vi "cDAQcoverterfilereader.vi"(8 "error in (no error)":errorcluster, 11 "name or relative path":string="Settings\\cDAQ\\converterSettings.txt") -> (0 "error out":errorcluster, 1 "Range":dbl[](array[numeric]), 2 "AI Max range of cDAQ":dbl[](array[numeric]), 3 "AI Min range of cDAQ":dbl[](array[numeric]), 5 "offset":dbl[](array[numeric]))   [LabVIEW 2019]
uses:
  <vilib>/Utility/file.llb/Read Delimited Spreadsheet (string).vi
panel:
  out "all rows":string[][](array[string])
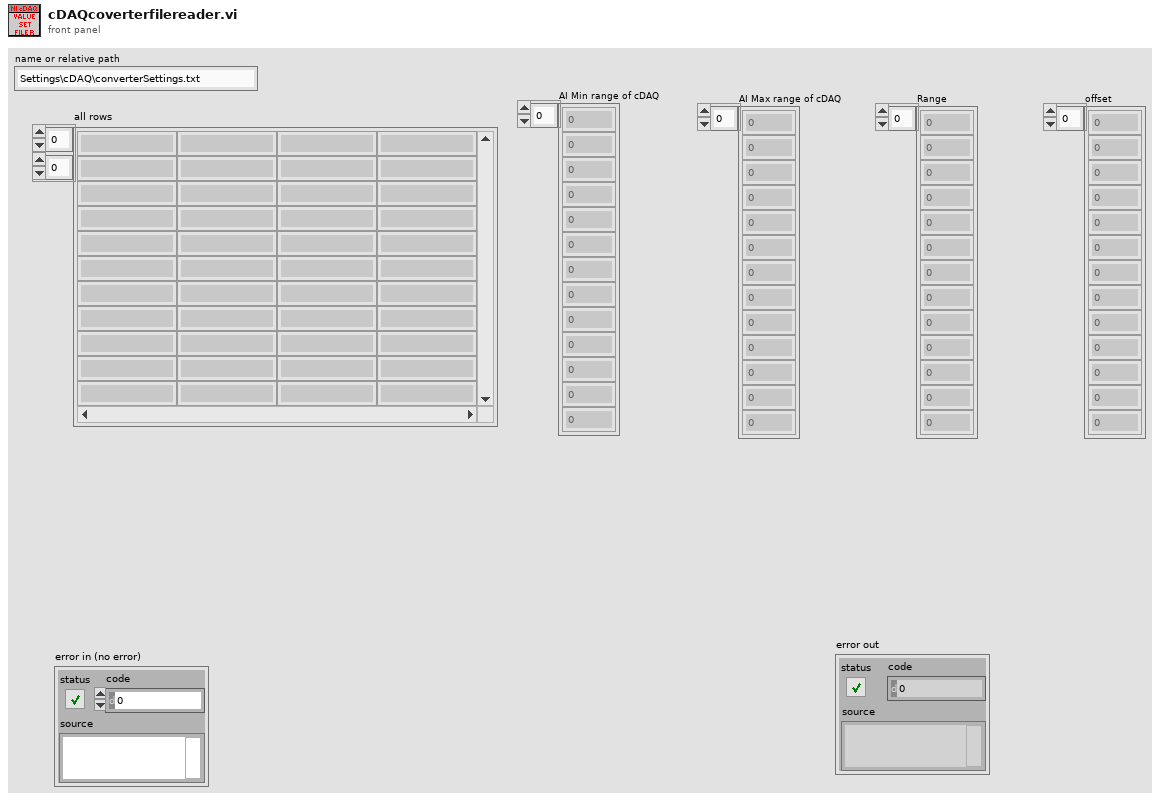
[diagram p1: front panel]
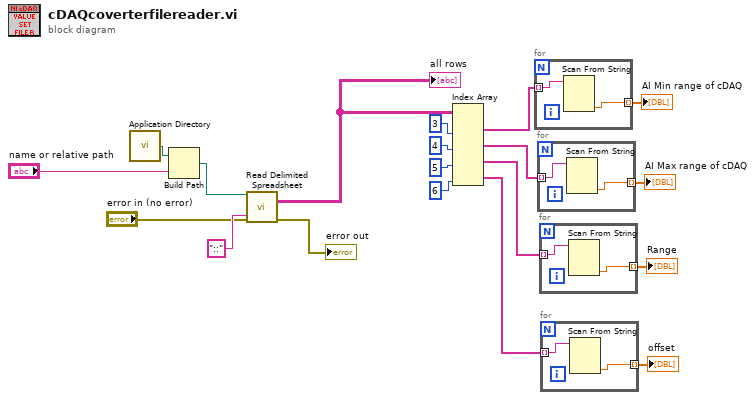
[diagram p0: block diagram]
diagram:
  n1 = call <vilib>:"Application Directory.vi"() -> ("Application Directory"=w19:path)
  n2 = Build Path(base path=w19, name or relative path="name or relative path") -> (appended path=w17:path)
  n3 = call-poly <vilib>:"Read Delimited Spreadsheet.vi"("file path (dialog if empty)"=w17, "error in (no error)"="error in (no error)", "delimiter (\\t)"="::" ("format (%.3f)")) -> ("all rows"=w15:string[][], "error out"=→"error out":errorcluster)  [unwired: 7 in, 4 out]
  "all rows" <- w15
  n4 = Index Array(array=w15, index (col) #1=3 ("disabled index (col)"), index (col) #2=4 ("index (col)"), index (col) #3=5 ("index (col)"), index (col) #4=6 ("index (col)")) -> (element #1=w9:string[], element #2=w8:string[], element #3=w7:string[], element #4=w1:string[])  [unwired: 4 in]
  n5 = for {
    tunnel: w9 -> [w21] mode=indexing
    tunnel: [w20] -> w6 mode=indexing
    n6 = Scan From String(input string=w21) -> (output 1=w20:dbl)  [unwired: 4 in, 3 out]
  }
  "AI Min range of cDAQ" <- w6
  n7 = for {
    tunnel: w8 -> [w23] mode=indexing
    tunnel: [w22] -> w5 mode=indexing
    n8 = Scan From String(input string=w23) -> (output 1=w22:dbl)  [unwired: 4 in, 3 out]
  }
  "AI Max range of cDAQ" <- w5
  n9 = for {
    tunnel: w7 -> [w25] mode=indexing
    tunnel: [w24] -> w4 mode=indexing
    n10 = Scan From String(input string=w25) -> (output 1=w24:dbl)  [unwired: 4 in, 3 out]
  }
  "Range" <- w4
  n11 = for {
    tunnel: w1 -> [w27] mode=indexing
    tunnel: [w26] -> w3 mode=indexing
    n12 = Scan From String(input string=w27) -> (output 1=w26:dbl)  [unwired: 4 in, 3 out]
  }
  "offset" <- w3
